vi "MakeNewExperiment.vi"(8 "error in (no error)":errorcluster, 11 "User Libraray in":path) -> (0 "error out":errorcluster, 3 "Created OK":bool)   [LabVIEW 2017]
uses:
  <userlib>/_OpenG.lib/file/file.llb/File Exists - Scalar__ogtk.vi
panel:
  out "User Libraray":path
  in  "btnCancel":bool
  in  "btnMake":bool
  in  "Experiment name (directory name)":string="MyExperiment"
  in  "From Template":i32(listbox)
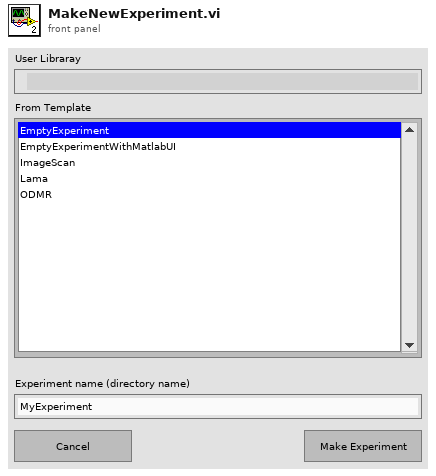
[diagram p1: front panel]
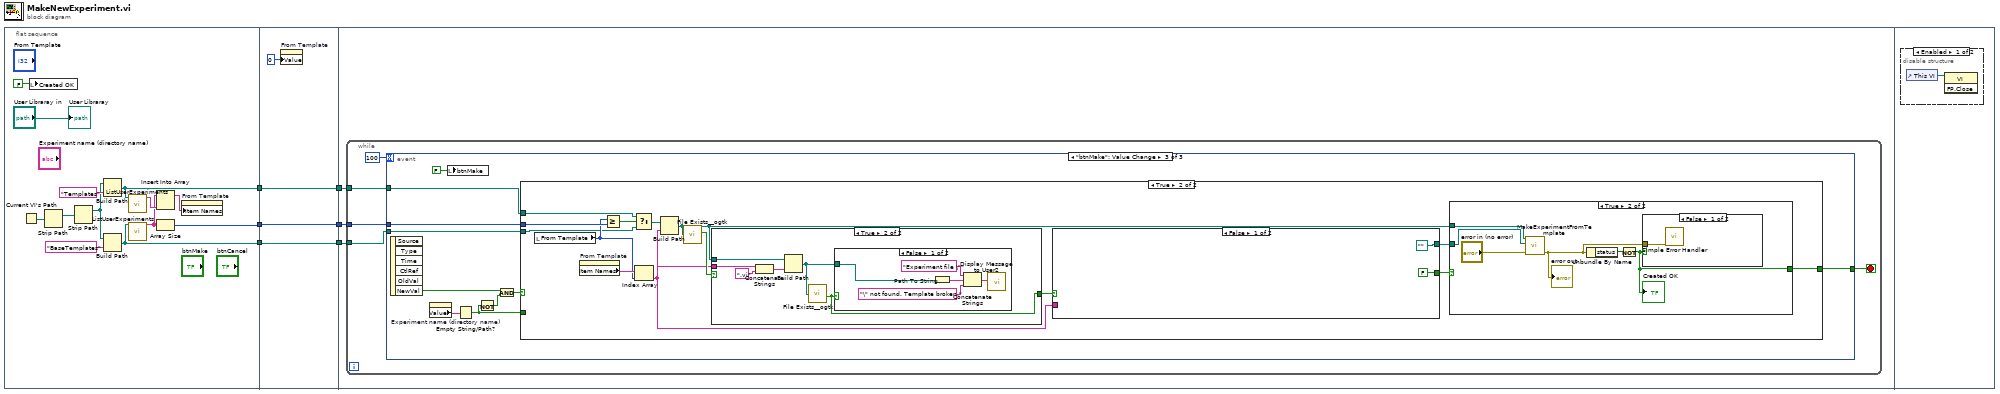
[diagram p0: block diagram]
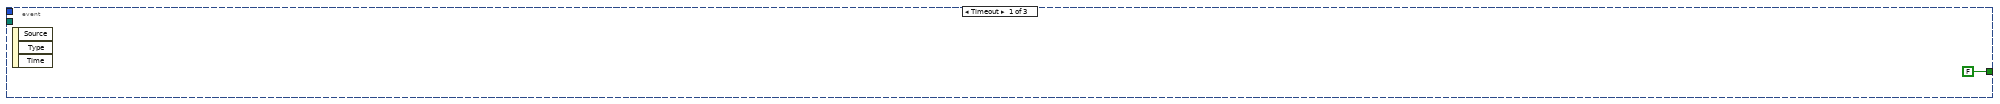
[diagram p2: hidden frame]
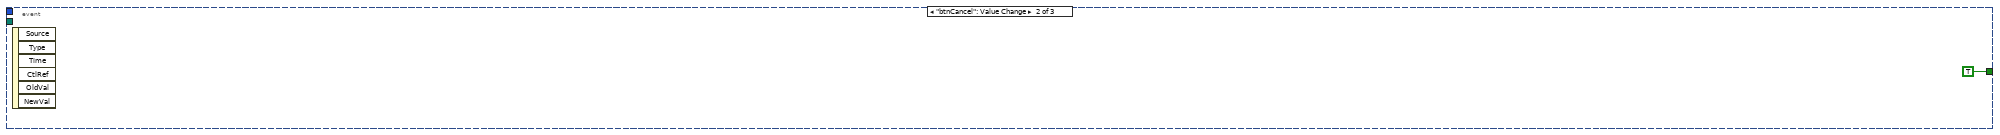
[diagram p3: hidden frame]
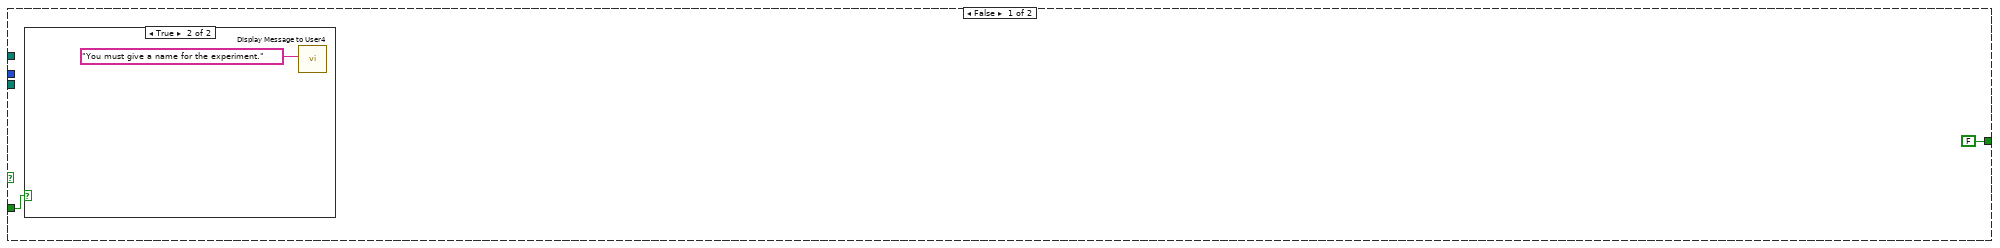
[diagram p4: hidden frame]
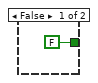
[diagram p6: hidden frame]
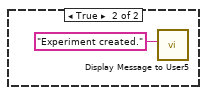
[diagram p7: hidden frame]
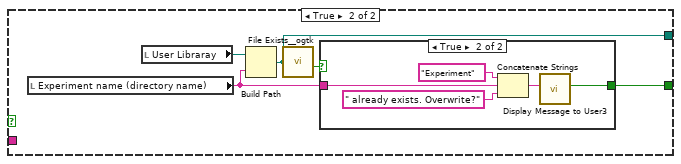
[diagram p8: hidden frame]
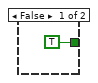
[diagram p9: hidden frame]
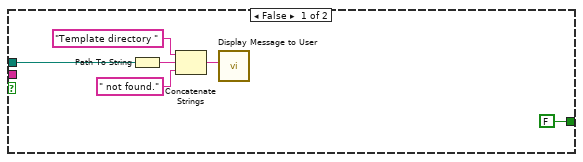
[diagram p10: hidden frame]
diagram:
  n1 = flat-sequence {
    tunnel: [w12] -> w6
    tunnel: [w11] -> w3
    tunnel: [w10] -> w1
    tunnel: w6 -> [w22]
    tunnel: [w22] -> w5
    tunnel: [w21] -> w4
    tunnel: w3 -> [w21]
    tunnel: [w20] -> w2
    tunnel: w1 -> [w20]
    tunnel: w5 -> [w26]
    tunnel: w4 -> [w25]
    tunnel: w2 -> [w24]
    frame #0 {
      n2 = Current VI's Path() -> (path=w18:path)
      n3 = local write "Created OK"(FALSE ("Created OK")) -> ()
      n4 = Strip Path(path=w18) -> (stripped path=w8:path)  [unwired: 1 out]
      n5 = Strip Path(path=w8) -> (stripped path=w7:path)  [unwired: 1 out]
      n6 = Build Path(base path=w7, name or relative path="Templates") -> (appended path=w10:path)
      n7 = Build Path(base path=w7, name or relative path="BaseTemplates") -> (appended path=w11:path)
      n8 = call "ListUserExperiments.vi"("Current user path"=w10) -> ("Sorted Array out"=w15:string[])  [unwired: 10 in]
      n9 = call "ListUserExperiments.vi"("Current user path"=w11) -> ("Sorted Array out"=w13:string[])  [unwired: 10 in]
      n10 = Insert Into Array(array=w13, new element=w15) -> (w14:string[])  [unwired: 1 in]
      n11 = Array Size(array=w13) -> (size(s)=w12:i32)
      n12 = property on="From Template" class="LstBox (strict)"("Item Names"=w14) -> ()  [unwired: 2 in, 2 out]
      "User Libraray" <- "User Libraray in"
    }
    frame #1 {
      n13 = property on="From Template" class="LstBox (strict)"("Value"=0 ("From Template")) -> ()  [unwired: 2 in, 2 out]
    }
    frame #2 {
      n14 = while {
        tunnel: w26 -> [w29]
        tunnel: w25 -> [w28]
        tunnel: w24 -> [w27]
        stop <- w31 stop-if-true
        n15 = event shown="[2] \"btnMake\": Value Change" {
          selector: _ -> [_ _ _]
          dyn-events: _ -> [_ _ _]
          timeout: 100 -> [_ _ _]
          tunnel: [FALSE TRUE w40] -> w31
          tunnel: w29 -> [_ _ w43]
          tunnel: w28 -> [_ _ w42]
          tunnel: w27 -> [_ _ w41]
          event Timeout {
            n16 = event-data() -> ()  [unwired: 1 in, 3 out]
          }
          event "btnCancel": Value Change {
            n17 = event-data() -> ()  [unwired: 1 in, 6 out]
          }
          event "btnMake": Value Change {
            n18 = event-data() -> ("NewVal"=w38:bool)  [unwired: 1 in, 5 out]
            n19 = property on="Experiment name (directory name)" class="Str"() -> ("Value"=w39:string)  [unwired: 2 in, 2 out]
            n20 = local write "btnMake"(FALSE ("btnMake")) -> ()
            n21 = Empty String/Path?(string/path=w39) -> (empty?=w35:bool)
            n22 = Not(x=w35) -> (.not. x?=w37:bool)
            n23 = And(x=w38, y=w37) -> (x .and. y?=w36:bool)
            n24 = case shown="True" w36 {
              tunnel: w43 -> [_ w60]
              tunnel: w42 -> [_ w55]
              tunnel: w41 -> [_ w56]
              tunnel: [FALSE w47] -> w40
              tunnel: w35 -> [w45 _]
              frame False {
                n25 = case shown="True" w45 {
                  frame False {
                  }
                  frame True {
                    n26 = call "Display Message to User4"("Message"="You must give a name for the experiment.") -> ()  [unwired: 9 in, 2 out]
                  }
                }
              }
              frame True {
                n27 = local read "From Template"() -> (w58:i32)
                n28 = property on="From Template" class="LstBox (strict)"() -> ("Item Names"=w59:string[])  [unwired: 2 in, 2 out]
                n29 = Greater Or Equal?(x=w58, y=w60) -> (x >= y?=w57:bool)
                n30 = Select(t=w56, s=w57, f=w55) -> (s? t:f=w54:path)
                n31 = Index Array(array=w59, index=w58) -> (element=w48:string)
                n32 = Build Path(base path=w54, name or relative path=w48) -> (appended path=w50:path)
                n33 = call-poly <userlib>:"File Exists__ogtk.vi"("file path"=w50) -> ("is directory"=w53:bool)  [unwired: 6 in, 1 out]
                n34 = case shown="True" w53 {
                  tunnel: w50 -> [w87 w91]
                  tunnel: w48 -> [_ w94]
                  tunnel: [FALSE ("exists") w90] -> w52
                  frame False {
                    n35 = Path To String(path=w87) -> (string=w86:string)
                    n36 = Concatenate Strings("Template directory " ("string"), w86, " not found." ("string")) -> (w84:string)
                    n37 = call "Display Message to User"("Message"=w84) -> ()  [unwired: 9 in, 2 out]
                  }
                  frame True {
                    n38 = Concatenate Strings(w94, ".vi" ("string")) -> (w92:string)
                    n39 = Build Path(base path=w91, name or relative path=w92) -> (appended path=w89:path)
                    n40 = call-poly <userlib>:"File Exists__ogtk.vi"("file path"=w89) -> ("exists"=w90:bool)  [unwired: 6 in, 1 out]
                    n41 = case shown="False" w90 {
                      tunnel: w89 -> [w96 _]
                      frame False {
                        n42 = Path To String(path=w96) -> (string=w95:string)
                        n43 = Concatenate Strings("Experiment file \"" ("string"), w95, "\" not found. Template broken." ("string")) -> (w97:string)
                        n44 = call "Display Message to User2"("Message"=w97) -> ()  [unwired: 9 in, 2 out]
                      }
                      frame True {
                      }
                    }
                  }
                }
                n45 = case shown="False" w52 {
                  tunnel: w48 -> [_ _]
                  tunnel: [FALSE ("Overwrite") w74] -> w51
                  tunnel: [path "" ("appended path") w73] -> w49
                  frame False {
                  }
                  frame True {
                    n46 = local read "Experiment name (directory name)"() -> (w72:string)
                    n47 = local read "User Libraray"() -> (w76:path)
                    n48 = Build Path(base path=w76, name or relative path=w72) -> (appended path=w73:path)
                    n49 = call-poly <userlib>:"File Exists__ogtk.vi"("file path"=w73) -> ("exists"=w75:bool)  [unwired: 6 in, 1 out]
                    n50 = case shown="True" w75 {
                      tunnel: w72 -> [_ w79]
                      tunnel: [TRUE ("Overwrite") w78] -> w74
                      frame False {
                      }
                      frame True {
                        n51 = Concatenate Strings("Experiment" ("string"), w79, " already exists. Overwrite?" ("string")) -> (w80:string)
                        n52 = call "Display Message to User3"("Message"=w80) -> ("Overwrite"=w78:bool)  [unwired: 9 in, 1 out]
                      }
                    }
                  }
                }
                n53 = case shown="True" w51 {
                  tunnel: w50 -> [_ w66]
                  tunnel: w49 -> [_ w65]
                  tunnel: [FALSE ("status") w63] -> w47
                  frame False {
                  }
                  frame True {
                    n54 = call "MakeExperimentFromTemplate.vi"("error in (no error)"="error in (no error)", "Target experiment directory"=w65, "Source template directory"=w66) -> ("error out"=w62:errorcluster)  [unwired: 8 in]
                    "error out" <- w62
                    n55 = Unbundle By Name(w62) -> ("status"=w64:bool)
                    n56 = Not(x=w64) -> (.not. x?=w63:bool)
                    "Created OK" <- w63
                    n57 = case shown="False" w63 {
                      tunnel: w62 -> [w68 _]
                      frame False {
                        n58 = call <vilib>:"Simple Error Handler.vi"("error in (no error)"=w68) -> ()  [unwired: 4 in, 5 out]
                      }
                      frame True {
                        n59 = call "Display Message to User5"("Message"="Experiment created.") -> ()  [unwired: 9 in, 2 out]
                      }
                    }
                  }
                }
              }
            }
          }
        }
      }
    }
    frame #3 {
      n60 = disable-structure shown="Enabled" {
        frame Enabled {
          n61 = control-ref of="This VI"() -> (w100:refnum<vi>)
          n62 = invoke class="VI" method="FP.Close"(reference=w100) -> ()  [unwired: 2 in, 3 out]
        }
        frame Disabled {
        }
      }
    }
  }
